vi "ECAT Download Error Handle.vi"(8 "error in":errorcluster) -> (0 "error out":errorcluster, 3 "Message output":string)   [LabVIEW 2019, in "SEECD System Explorer.lvlib"]
uses:
  SEECD System Explorer.lvlib
  <vilib>/Utility/error.llb/DialogType.ctl
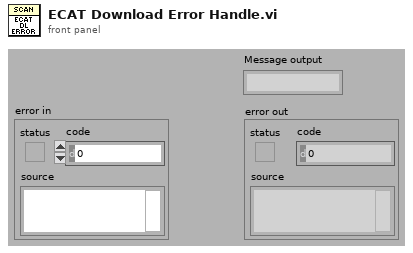
[diagram p1: front panel]
types:
  T1 = typedef "DialogType.ctl" = u16
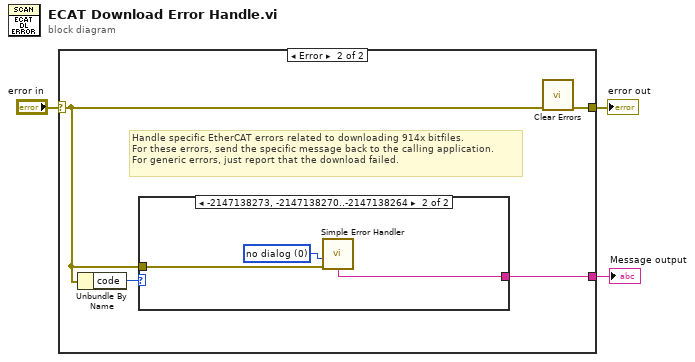
[diagram p0: block diagram]
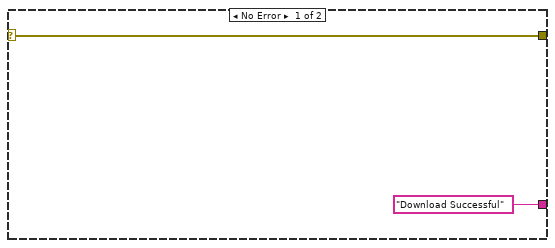
[diagram p2: hidden frame]
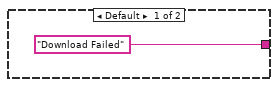
[diagram p3: hidden frame]
diagram:
  n1 = case shown="Error" "error in" {
    selector: "error in" -> [w5 w7]
    tunnel: [w5 w9] -> w3
    tunnel: ["Download Successful" ("message") w6] -> w1
    frame No Error {
    }
    frame Error {
      # "Handle specific EtherCAT errors related to downloading 914x bitfiles.\nFor these errors, send the specific message back to the calling application.\nFor generic errors, just report that the download failed."
      n2 = Unbundle By Name(w7) -> ("code"=w8:i32)
      n3 = case shown="-2147138273, -2147138270..-2147138264" w8 {
        tunnel: w7 -> [_ w13]
        tunnel: ["Download Failed" ("message") w11] -> w6
        frame Default {
        }
        frame -2147138273, -2147138270..-2147138264 {
          w12 = T1 0 items=["no dialog", "OK message", "continue or stop message", "OK message + warnings", "continue/stop + warnings"] ("type of dialog (OK msg:1)")
          n4 = call <vilib>:"Simple Error Handler.vi"("type of dialog (OK msg:1)"=w12, "error in (no error)"=w13) -> ("message"=w11:string)  [unwired: 3 in, 4 out]
        }
      }
      n5 = call <vilib>:"Clear Errors.vi"("error in (no error)"=w7) -> ("error out"=w9:errorcluster)  [unwired: 1 in, 5 out]
    }
  }
  "error out" <- w3
  "Message output" <- w1
